vi "Actor Core.vi"(8 "error in":errorcluster, 11 "File Actor in":refnum<class "File Actor.lvclass">) -> (0 "error out":errorcluster, 3 "Actor out":refnum<class "Actor.lvclass">)   [LabVIEW 2017, in "File Library.lvlib" / "File Actor.lvclass"]
doc: "(<B>Filename</B>: Actor Framework.lvlib:Actor.lvclass:Actor Core.vi)\n\nReceives messages to the actor, reacts to them, and initiates any error handling that may shut the actor down.\n\nDescendant classes may override this VI to append parallel tasks for the actor to complete while it handles messages. Overrides use the Call Parent Method node."
uses:
  File Actor.lvclass
  C:/Program Files (x86)/National Instruments/LabVIEW 2017/vi.lib/ActorFramework/Actor/Actor.lvclass
  <vilib>/ActorFramework/Actor/Actor.lvclass
  <vilib>/ActorFramework/Actor/Actor.lvclass/Actor.ctl
  <vilib>/ActorFramework/Message Enqueuer/Message Enqueuer.lvclass/Message Enqueuer.ctl
  File Actor.lvclass/File Actor.ctl
  Messages/To/Check File Size MSG/Check File Size MSG.lvclass
  C:/Program Files (x86)/National Instruments/LabVIEW 2017/vi.lib/ActorFramework/Message/Message.lvclass
  <vilib>/ActorFramework/Message Enqueuer/Init from Existing Queue.vi
  <vilib>/ActorFramework/Message Priority Queue/Priority Enqueue.vi
  <vilib>/MSR Consulting, LLC/General Reuse/SuperActor/SuperActor.lvclass
  <vilib>/ActorFramework/Message Enqueuer/Message Enqueuer.lvclass
  <vilib>/MSR Consulting, LLC/General Reuse/Command/Command.lvclass
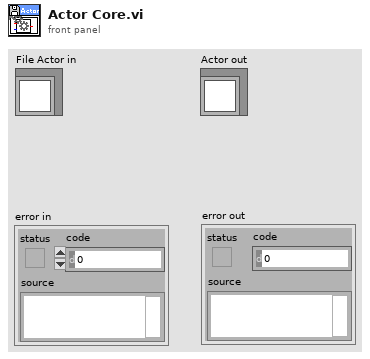
[diagram p1: front panel]
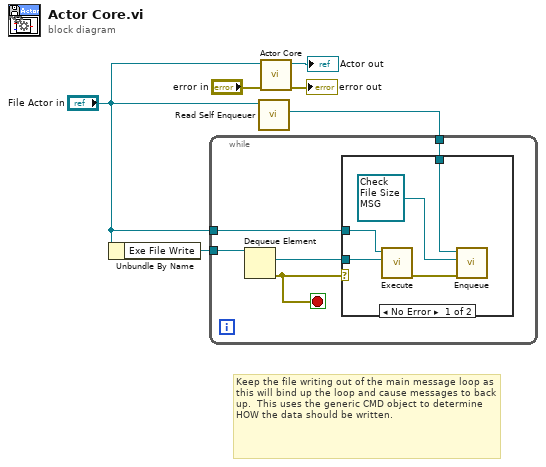
[diagram p0: block diagram]
diagram:
  # "Keep the file writing out of the main message loop as this will bind up the loop and cause messages to back up.  This uses the generic CMD object to determine HOW the data should be written."
  n1 = Unbundle By Name("File Actor in") -> ("Exe File Write"=w1:refnum<queue>)
  n2 = call <vilib>:"Read Self Enqueuer.vi"("Actor"="File Actor in") -> ("Self Enqueuer"=w2:refnum<class "Message Enqueuer.lvclass">)  [unwired: 10 in]
  n3 = while {
    tunnel: w1 -> [w11]
    tunnel: "File Actor in" -> [w8]
    tunnel: w2 -> [w7]
    stop <- w10 stop-if-true
    n4 = Dequeue Element(queue=w11) -> (element=w9:refnum<class "Command.lvclass">, error out=w10:errorcluster)  [unwired: 2 in, 2 out]
    n5 = case shown="No Error" w10 {
      tunnel: w9 -> [w16 _]
      tunnel: w8 -> [w15 _]
      tunnel: w7 -> [w14 _]
      frame No Error {
        n6 = call <vilib>:"Execute.vi"("Command in"=w16, "Object In"=w15) -> ("error out"=w12:errorcluster)  [unwired: 8 in, 1 out]
        n7 = call <vilib>:"Enqueue.vi"("error in (no error)"=w12, "Message"=refnum<class "Check File Size MSG.lvclass"> refnum ("File Library.lvlib:Check File Size MSG"), "Message Enqueuer in"=w14) -> ()  [unwired: 7 in, 2 out]
      }
      frame Error {
      }
    }
  }
  n8 = call-parent "Actor Core.vi"("error in"="error in", "Actor in"="File Actor in") -> ("error out"=→"error out":errorcluster, "Actor out"=→"Actor out":refnum<class "Actor.lvclass">)  [unwired: 8 in]
